vi "Get Channel Identifiers.vi"(8 "error in":errorcluster, 11 "DAQmx Base Configure Strategy in":refnum<class "DAQmx Base Configure Strategy.lvclass">) -> (0 "error out":errorcluster, 2 "Channel Identifiers":string[](array[string]), 3 "DAQmx Base Configure Strategy out":refnum<class "DAQmx Base Configure Strategy.lvclass">)   [LabVIEW 2024, in "DAQmx Base Configure Strategy.lvclass"]
uses:
  DAQmx Base Configure Strategy.lvclass
  DAQmx Base Configure Strategy.lvclass/DAQmx Base Configure Strategy.ctl
  <resource>/objmgr/daqmx.rc
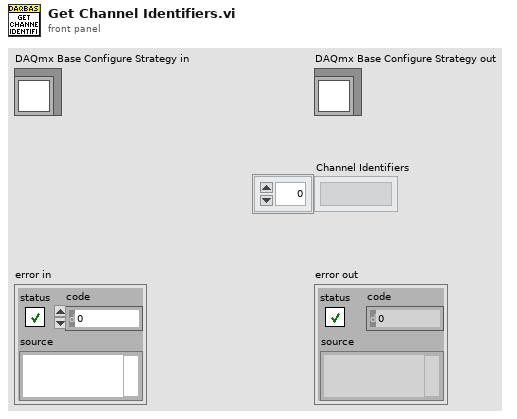
[diagram p1: front panel]
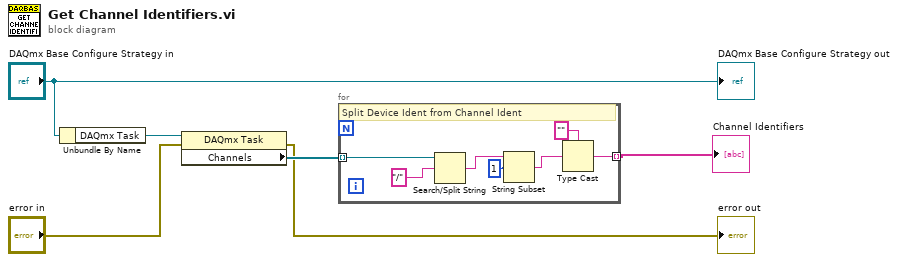
[diagram p0: block diagram]
diagram:
  n1 = Unbundle By Name("DAQmx Base Configure Strategy in") -> ("DAQmx Task"=w5:refnum<k21>)
  n2 = property class="DAQmx Task"(reference=w5, error in="error in") -> (error out=→"error out":errorcluster, "Channels"=w3:refnum<k21>[])  [unwired: 1 out]
  n3 = for {
    tunnel: w3 -> [w11] mode=indexing
    tunnel: [w12] -> w2 mode=indexing
    # "Split Device Ident from Channel Ident"
    n4 = Search/Split String(string=w11, search string/char (-)="/") -> (match + rest of string=w8:string)  [unwired: 1 in, 2 out]
    n5 = String Subset(string=w8, offset (0)=1) -> (substring=w7:string)  [unwired: 1 in]
    n6 = Type Cast(type="", x=w7) -> (*(type *) &x=w12:string)
  }
  "Channel Identifiers" <- w2
  "DAQmx Base Configure Strategy out" <- "DAQmx Base Configure Strategy in"
